vi "Measurement Query.vi"(0 "RedPitaya connection in":refnum<k5>, 2 "Query setting":u16(ring) items=["Vpp", "Mean voltage", "Max voltage", "Min voltage", "Signal frequency", "Signal period", "Duty cycle"], 5 "error in":errorcluster, 8 "Channel #":u16(ring)=1 items=["Channel 1"=1, "Channel 2"=2], 12 "timeout ms (2000)":i32=2000) -> (14 "RedPitaya connection out":refnum<k5>, 16 "Output string":string, 19 "error out":errorcluster)   [LabVIEW 2010, in "RedPitaya.lvlib"]
doc: "Returns specific information about signal measurement from Red Pitaya."
uses:
  RedPitaya.lvlib
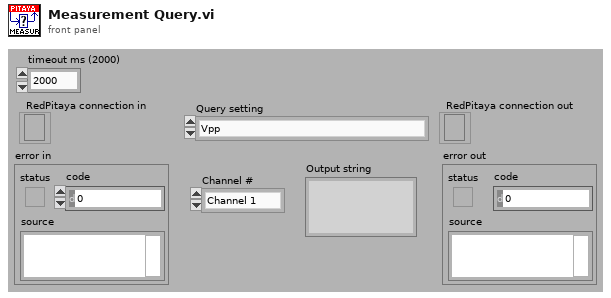
[diagram p1: front panel]
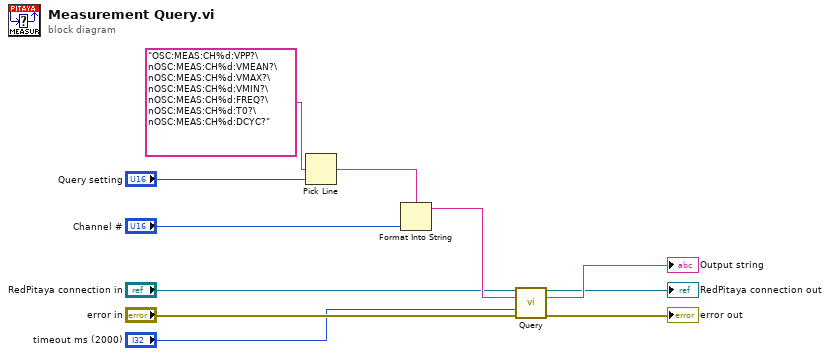
[diagram p0: block diagram]
diagram:
  n1 = Pick Line(multi-line string="OSC:MEAS:CH%d:VPP?\nOSC:MEAS:CH%d:VMEAN?\nOSC:MEAS:CH%d:VMAX?\nOSC:MEAS:CH%d:VMIN?\nOSC:MEAS:CH%d:FREQ?\nOSC:MEAS:CH%d:T0?\nOSC:MEAS:CH%d:DCYC?", line index="Query setting") -> (output string=w7:string)  [unwired: 1 in]
  n2 = Format Into String(format string=w7, "Channel #") -> (resulting string=w9:string)  [unwired: 2 in, 1 out]
  n3 = call "Query.vi"("RedPitaya connection in"="RedPitaya connection in", "SCPI Query"=w9, "timeout ms (2000)"="timeout ms (2000)", "error in"="error in") -> ("RedPitaya connection out"=→"RedPitaya connection out":refnum<k5>, "data out"=→"Output string":string, "error out"=→"error out":errorcluster)  [unwired: 9 in]
